vi "Triangular CDF.vi"(8 "xmax":dbl=1.0, 9 "xmode":dbl=nan, 10 "xmin":dbl, 11 "x":dbl=0.5) -> (0 "error":i32, 3 "cdf(x)":dbl=0.5)   [LabVIEW 2017, in "NI_Gmath.lvlib"]
doc: "Computes the continuous cumulative distribution function (CDF), or the probability that the random variate X, where X describes the selected distribution type, has a value less than or equal to <B>x</B>. You must manually select the polymorphic instance to use."
uses:
  NI_Gmath.lvlib
  st_error_code.ctl
panel:
  # "Triangular CDF"
  # "NaN maps to \n(xmax-xmin)/2"
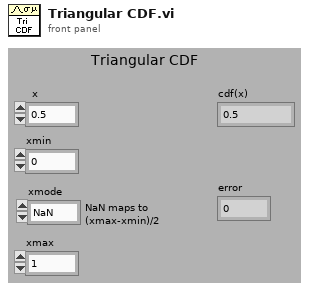
[diagram p1: front panel]
types:
  T1 = typedef "NI_Gmath.lvlib/st_error_code.ctl" = i32
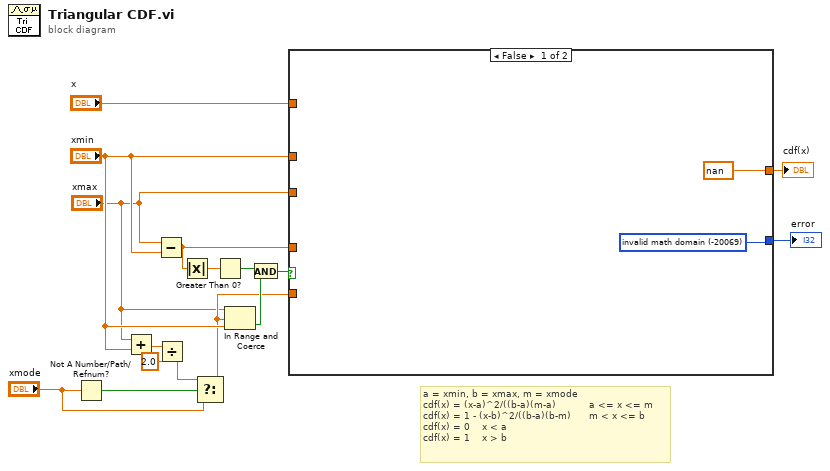
[diagram p0: block diagram]
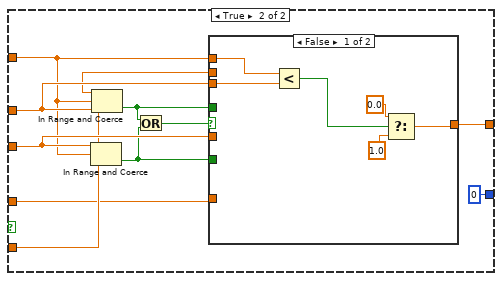
[diagram p2: hidden frame]
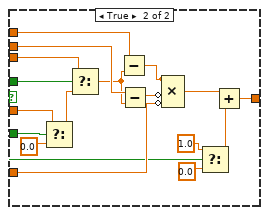
[diagram p3: hidden frame]
diagram:
  # "a = xmin, b = xmax, m = xmode\ncdf(x) = (x-a)^2/((b-a)(m-a)           a <= x <= m\ncdf(x) = 1 - (x-b)^2/((b-a)(b-m)      m < x <= b\ncdf(x) = 0    x < a\ncdf(x) = 1    x > b"
  n1 = Not A Number/Path/Refnum?(number/path/refnum="xmode") -> (NaN/Path/Refnum?=w5:bool)
  n2 = Add(x="xmax", y="xmin") -> (x+y=w8:dbl)
  n3 = Subtract(x="xmax", y="xmin") -> (x-y=w10:dbl)
  n4 = Divide(x=w8, y=2.0) -> (x/y=w6:dbl)
  n5 = Absolute Value(x=w10) -> (abs(x)=w15:dbl)
  n6 = Select(t=w6, s=w5, f="xmode") -> (s? t:f=w2:dbl)
  n7 = Greater Than 0?(x=w15) -> (x > 0?=w12:bool)
  n8 = In Range and Coerce(upper limit="xmax", x=w2, lower limit="xmin") -> (In Range?=w3:bool)  [unwired: 1 out]
  n9 = And(x=w12, y=w3) -> (x .and. y?=w11:bool)
  n10 = case shown="False" w11 {
    tunnel: "x" -> [_ w25]
    tunnel: "xmin" -> [_ w27]
    tunnel: w10 -> [_ w23]
    tunnel: [nan w22] -> w14
    tunnel: [w17 0] -> w13
    tunnel: w2 -> [_ w24]
    tunnel: "xmax" -> [_ w26]
    frame False {
      w17 = T1 -20069 items=["invalid math domain"=-20069, "Fourier interpolation size m >= n"=-20070, "empty array"=-20003] ("stat interp error code")
    }
    frame True {
      n11 = In Range and Coerce(upper limit=w26, x=w25, lower limit=w24) -> (In Range?=w20:bool)  [unwired: 1 out]
      n12 = In Range and Coerce(upper limit=w24, x=w25, lower limit=w27) -> (In Range?=w21:bool)  [unwired: 1 out]
      n13 = Or(x=w21, y=w20) -> (x .or. y?=w19:bool)
      n14 = case shown="False" w19 {
        tunnel: w27 -> [w34 w51]
        tunnel: w26 -> [_ w50]
        tunnel: w25 -> [w31 w49]
        tunnel: w24 -> [_ w48]
        tunnel: w23 -> [_ w47]
        tunnel: [w29 w46] -> w22
        tunnel: w21 -> [_ w45]
        tunnel: w20 -> [_ w40]
        frame False {
          n15 = Less?(x=w31, y=w34) -> (x < y?=w32:bool)
          n16 = Select(t=0.0, s=w32, f=1.0 ("t")) -> (s? t:f=w29:dbl)
        }
        frame True {
          n17 = Select(t=w50, s=w40, f=0.0) -> (s? t:f=w44:dbl)
          n18 = Select(t=w51, s=w45, f=w44) -> (s? t:f=w35:dbl)
          n19 = Subtract(x=w49, y=w35) -> (x-y=w42:dbl)
          n20 = Subtract(x=w48, y=w35) -> (x-y=w41:dbl)
          n21 = Compound Arithmetic op=MULTIPLY(w42, w42, invert w41, invert w47) -> (w37:dbl)
          n22 = Select(t=1.0, s=w40, f=0.0 ("t")) -> (s? t:f=w36:dbl)
          n23 = Add(x=w37, y=w36) -> (x+y=w46:dbl)
        }
      }
    }
  }
  "cdf(x)" <- w14
  "error" <- w13
